vi "LED (SubVI).vi"(10 "state":u8, 11 "ID":u8) -> (3 "result string":string)   [LabVIEW 2017]
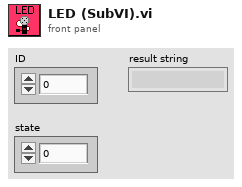
[diagram p1: front panel]
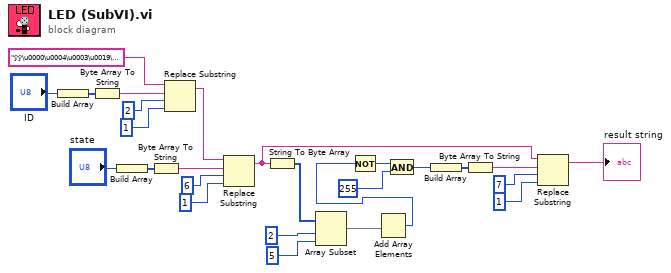
[diagram p0: block diagram]
diagram:
  n1 = Build Array("ID") -> (w4:u8[])
  n2 = Byte Array To String(unsigned byte array=w4) -> (string=w2:string)
  n3 = Build Array("state") -> (w9:u8[])
  n4 = Byte Array To String(unsigned byte array=w9) -> (string=w7:string)
  n5 = Replace Substring(2:1 ("length (len. of substring)"), 3:2 ("offset (0)"), 4:w2, 5:"ÿÿ\u0000\u0004\u0003\u0019\u0000\u0000" ("string")) -> (1:w12:string)  [unwired: 1 out]
  n6 = Replace Substring(2:1 ("length (len. of substring)"), 3:6 ("offset (0)"), 4:w7, 5:w12) -> (1:w20:string)  [unwired: 1 out]
  n7 = String To Byte Array(string=w20) -> (unsigned byte array=w22:u8[])
  n8 = Array Subset(array=w22, index=2, length=5) -> (w25:u8[])
  n9 = Add Array Elements(numeric array=w25) -> (sum=w26:u8)
  n10 = Not(x=w26) -> (.not. x?=w13:u8)
  n11 = And(x=w13, y=u8 255) -> (x .and. y?=w19:u8)
  n12 = Build Array(w19) -> (w16:u8[])
  n13 = Byte Array To String(unsigned byte array=w16) -> (string=w15:string)
  n14 = Replace Substring(2:1 ("length (len. of substring)"), 3:7 ("offset (0)"), 4:w15, 5:w20) -> (1:→"result string":string)  [unwired: 1 out]
